vi "Preview One Sample.vi"(7 "Host Resources":T4, 9 "Channel to preview":i32, 11 "Channel Settings":T1[](array[typedef])) -> (1 "Channel to preview out":i32, 2 "Waveform":waveform(dbl), 3 "Channel Settings out":T1[](array[typedef]))   [LabVIEW 2021, in "Acquisition.lvlib"]
doc: "Isolate the 'Channel to preview' from 'Channel Settings' and return one measurement."
uses:
  Acquisition.lvlib
  Channel Settings.ctl
  IO Device.ctl
  Sensor Type.ctl
  Host Resources.ctl
  Host Software Package.ctl
  Host IO Resource.ctl
  API Call.ctl
  support/Message Queue/Message Cluster.ctl
  support/Message Queue/Message Queue.lvlib
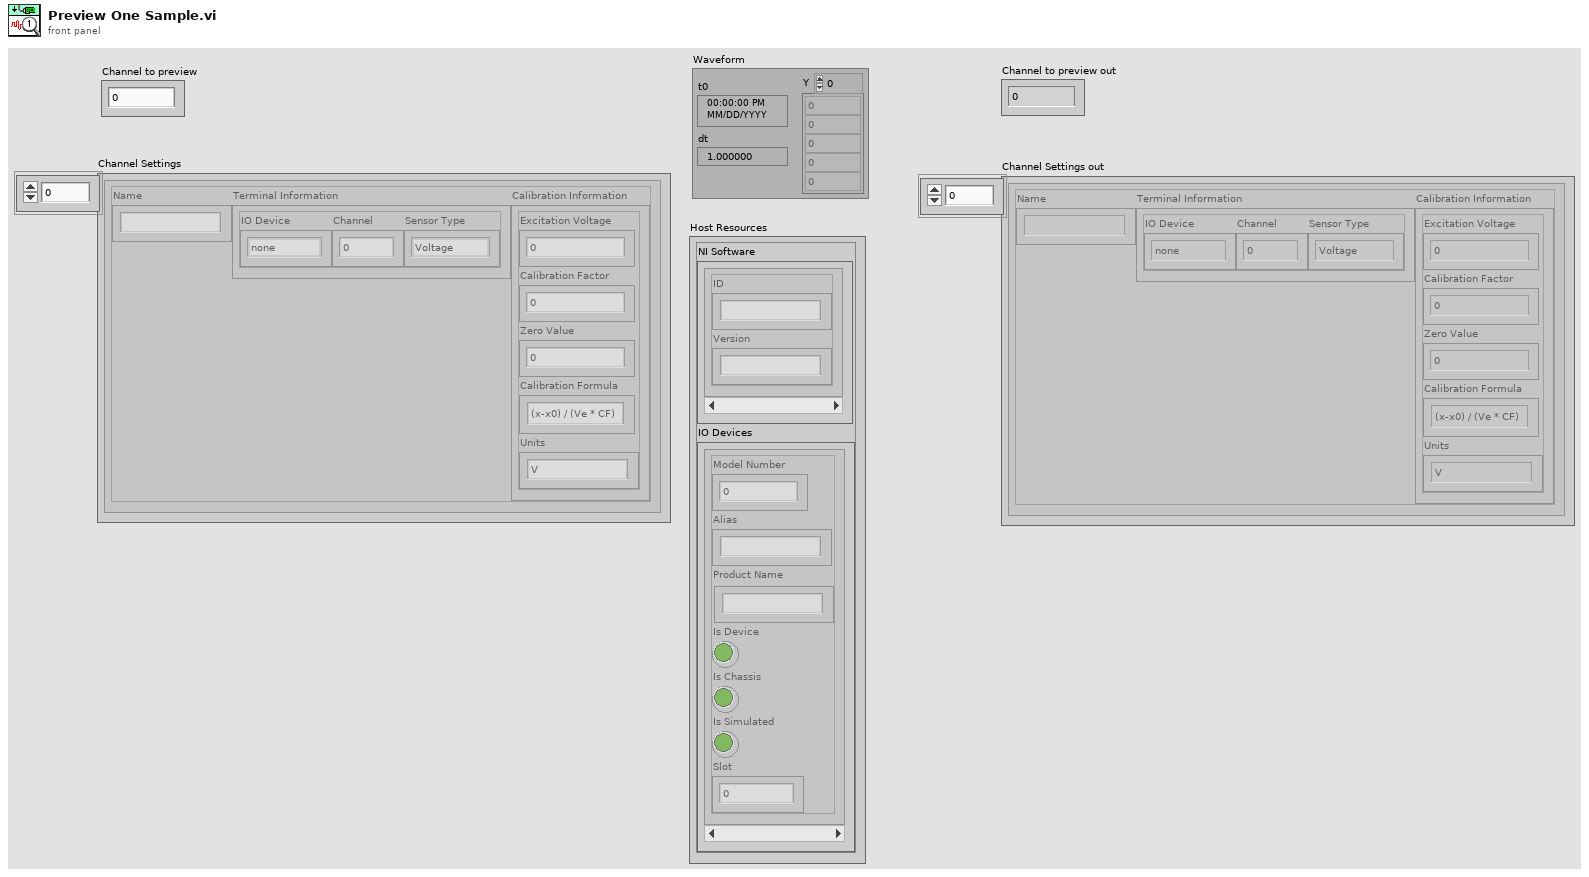
[diagram p1: front panel]
types:
  T1 = typedef "Acquisition.lvlib/Channel Settings.ctl" = cluster{"Name":string, "Terminal Information":cluster{"IO Device":T2, "Channel":i32, "Sensor Type":T3}, "Calibration Information":cluster{"Excitation Voltage":dbl, "Calibration Factor":dbl, "Zero Value":dbl, "Calibration Formula":string, "Units":string}}
  T2 = typedef "Acquisition.lvlib/IO Device.ctl" = enum16{"none", "9219", "9401"}
  T3 = typedef "Acquisition.lvlib/Sensor Type.ctl" = enum16{"Voltage", "Load", "Pressure", "Encoder"}
  T4 = typedef "Acquisition.lvlib/Host Resources.ctl" = cluster{"NI Software":T5[], "IO Devices":T6[]}
  T5 = typedef "Acquisition.lvlib/Host Software Package.ctl" = cluster{"ID":string, "Version":string}
  T6 = typedef "Acquisition.lvlib/Host IO Resource.ctl" = cluster{"Model Number":u32, "Alias":string, "Product Name":string, "Is Device":bool, "Is Chassis":bool, "Is Simulated":bool, "Slot":i32}
  T7 = typedef "Acquisition.lvlib/API Call.ctl" = enum16{"On Start", "Acquire", "On Stop", "Preview"}
  T8 = typedef "Acquisition.lvlib/Hardware Configuration.ctl" = cluster{"Channel Settings":T1[], "Sensor Intervals":T9[], "Sensor Token":T11, "IO Context":T12}
  T9 = typedef "Interval Timer.lvlib/Repeat Interval.ctl" = cluster{"Interval":T10, "Count":i32}
  T10 = typedef "Interval Timer.lvlib/Interval Length.ctl" = enum16{"Manual control", "1 second", "10 seconds", "30 seconds", "60 seconds", "600 seconds", "1200 seconds", "3600 seconds"}
  T11 = typedef "Interval Timer.lvlib/Interval Token.ctl" = cluster{"Next reading in ms":u32, "Interval Index":i32, "Interval Occurrence":i32}
  T12 = typedef "Acquisition.lvlib/IO Context.ctl" = cluster{"API":T13, "API Wire":variant}
  T13 = typedef "Acquisition.lvlib/IO API.ctl" = enum16{"Simulated", "DAQmx"}
  T14 = typedef "Acquisition.lvlib/Acquired Data.ctl" = cluster{"Waveform Array":waveform(dbl)[]}
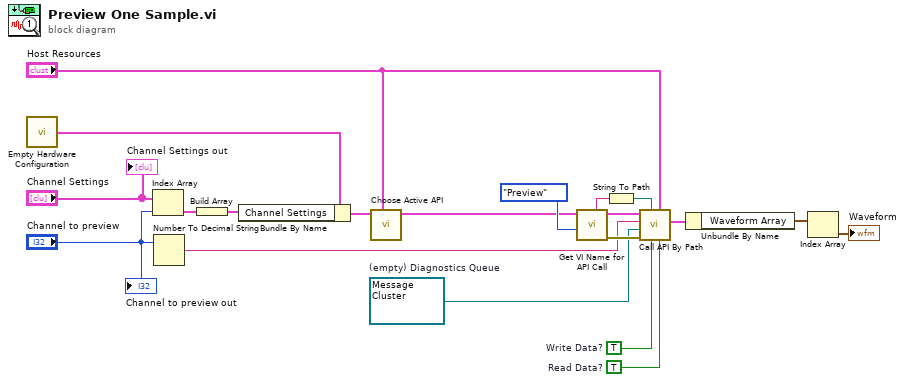
[diagram p0: block diagram]
diagram:
  w1 = refnum<queue> refnum  # (empty) Diagnostics Queue
  w7 = TRUE  # Write Data?
  w15 = TRUE  # Read Data?
  n1 = call "Empty Hardware Configuration.vi"() -> ("Hardware Configuration"=w14:T8)
  n2 = Index Array(array="Channel Settings", index="Channel to preview") -> (element=w12:T1)
  n3 = Number To Decimal String(number="Channel to preview") -> (decimal integer string=w3:string)  [unwired: 1 in]
  n4 = Build Array(w12) -> (w11:T1[])
  n5 = Bundle By Name(cluster=w14, "Channel Settings"=w11) -> (w5:T8)
  n6 = call "Choose Active API.vi"("Host Resources"="Host Resources", "Hardware Configuration in"=w5) -> ("Hardware Configuration out"=w4:T8)  [unwired: 9 in]
  n7 = call "Get VI Name for API Call.vi"("API Call"=API_Call."Preview", "Hardware Configuration in"=w4) -> ("error out"=w18:errorcluster, "Hardware Configuration out"=w17:T8, "VI Name"=w19:string)  [unwired: 7 in]
  n8 = String To Path(string=w19) -> (path=w20:path)
  n9 = call "Call API By Path.vi"("Read Data? (F)"=w15, "Host Resources"="Host Resources", "Write Data? (F)"=w7, "vi path"=w20, "error in"=w18, "Diagnostics Queue"=w1, "Generated Data"=w3, "Hardware Configuration in"=w17) -> ("Acquired Data"=w10:T14)  [unwired: 1 in, 2 out]
  n10 = Unbundle By Name(w10) -> ("Waveform Array"=w9:waveform(dbl)[])
  n11 = Index Array(array=w9) -> (element=→"Waveform":waveform(dbl))  [unwired: 1 in]
  "Channel Settings out" <- "Channel Settings"
  "Channel to preview out" <- "Channel to preview"
